vi "Save Sequence to file.vi"(8 "error in (no error)":errorcluster, 9 "Timing\ndelay":u32[](array[numeric]) min=1 max=255 step=1, 10 "Sequence":bool[][](array[boolean]), 11 "Sequence file path\n(file dialog if empty)":path=path "D:/martin/QPsw - github/QuPMX/seqtest") -> (0 "error out":errorcluster)   [LabVIEW 2020, in "QuPMXdriver.lvlib"]
doc: "Save sequences represented as bytes into a simple tab delimited text file."
uses:
  QuPMXdriver.lvlib
  <vilib>/Utility/file.llb/Write Delimited Spreadsheet (string).vi
  <vilib>/Utility/file.llb/Write Delimited Spreadsheet (I64).vi
panel:
  # "Slave index"
  # "1              2               3              4                5               6"
  # "Channel index"
  # "1     2       3      4       5      6      7       8      9     10     11    12"
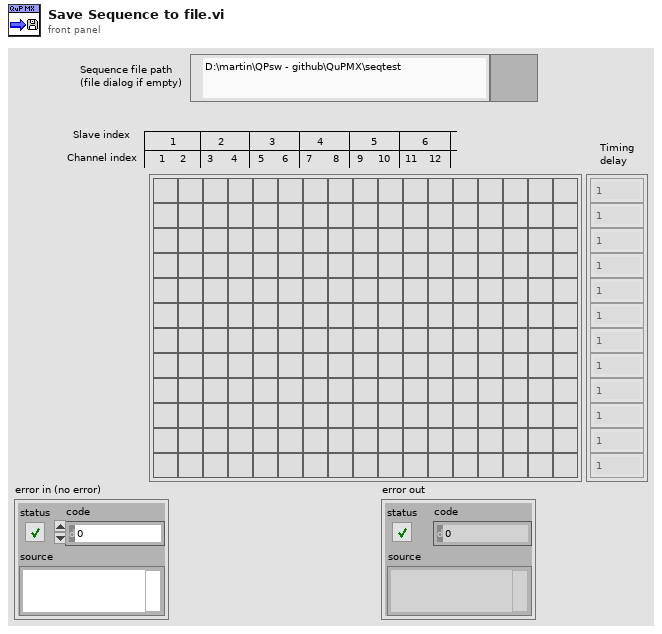
[diagram p1: front panel]
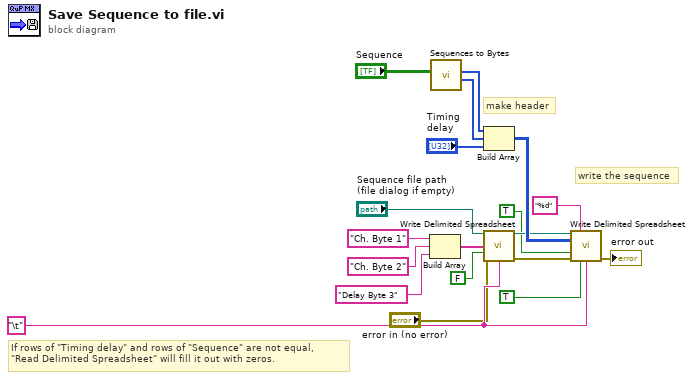
[diagram p0: block diagram]
diagram:
  w19 = "\t" ("delimiter (\\t)")
  # "write the sequence"
  # "make header"
  # "If rows of \"Timing delay\" and rows of \"Sequence\" are not equal, \n\"Read Delimited Spreadsheet\" will fill it out with zeros."
  n1 = Build Array("Ch. Byte 1" ("string"), "Ch. Byte 2" ("string"), "Delay Byte 3" ("string")) -> (w11:string[])
  n2 = call "Sequences to Bytes.vi"("Channel states"="Sequence") -> ("Ch. bytes 2"=w6:u8[], "Ch. bytes 1"=w7:u8[])  [unwired: 9 in]
  n3 = Build Array(w7, w6, "Timing\ndelay") -> (w16:u32[][])
  n4 = call-poly <vilib>:"Write Delimited Spreadsheet.vi"("file path (dialog if empty)"="Sequence file path\n(file dialog if empty)", "1D data"=w11, "append to file? (new file:F)"=FALSE, "error in (no error)"="error in (no error)", "delimiter (\\t)"=w19) -> ("new file path (Not A Path if cancelled)"=w15:path, "error out"=w12:errorcluster)  [unwired: 9 in]
  n5 = call-poly <vilib>:"Write Delimited Spreadsheet.vi"("file path (dialog if empty)"=w15, "format (%d)"="%d", "2D data"=w16, "append to file? (new file:F)"=TRUE, "error in (no error)"=w12, "transpose? (no:F)"=TRUE, "delimiter (\\t)"=w19) -> ("error out"=→"error out":errorcluster)  [unwired: 7 in, 1 out]
